vi "Send Event.vi"(10 "Data":variant, 11 "Modbus Shortcut":T1) -> ()   [LabVIEW 2020, in "Modbus.lvlib" / "Modbus.lvclass"]
uses:
  Modbus.lvclass
  Modbus Control Shortcut.ctl
  Modbus Channel Type.ctl
  Packed Libraries/Messaging.lvlibp/Message Cluster.ctl
  Packed Libraries/Messaging.lvlibp
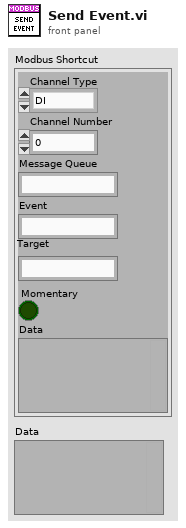
[diagram p1: front panel]
types:
  T1 = typedef "Modbus.lvlib/Modbus.lvclass/Modbus Control Shortcut.ctl" = cluster{"Channel Type":T2, "Channel Number":u8, "Message Queue":string, "Event":string, "Target":string, "Momentary":bool, "Data":variant}
  T2 = typedef "Modbus.lvlib/Modbus.lvclass/Modbus Channel Type.ctl" = enum16{"DI", "AI"}
  T3 = typedef "Messaging.lvlibp/Message Cluster.ctl" = cluster{"Event":string, "Source":string, "Target":string, "Data":variant}
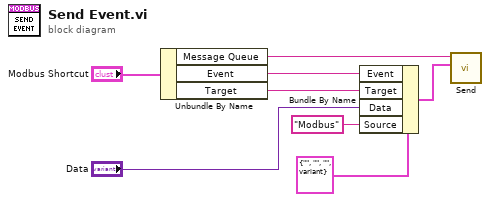
[diagram p0: block diagram]
diagram:
  n1 = Unbundle By Name("Modbus Shortcut") -> ("Message Queue"=w8:string, "Event"=w5:string, "Target"=w4:string)
  n2 = Bundle By Name(cluster=T3 {"Event"="", "Source"="", "Target"="", "Data"=variant} ("Message"), "Event"=w5, "Target"=w4, "Data"="Data", "Source"="Modbus") -> (w6:T3)
  n3 = call "Send.vi"("Message"=w6, "Queue Name"=w8) -> ()  [unwired: 9 in, 1 out]
